vi "Read Data as Bytes.vi"(7 "Read Image Size (Default: T)":bool=TRUE, 8 "error in (no error)":errorcluster, 11 "Buffer in":refnum<class "Buffer.lvclass">) -> (0 "error out":errorcluster, 1 "Image Size":T1, 2 "Data":u8[](array[numeric]), 3 "Buffer":refnum<class "Buffer.lvclass">)   [LabVIEW 2020, in "Buffer.lvclass"]
uses:
  Buffer.lvclass
  Image Size.ctl
  Buffer.lvclass/Buffer.ctl
  GetBufferImageDimensions.vi
  <vilib>/Utility/error.llb/Error Cluster From Error Code.vi
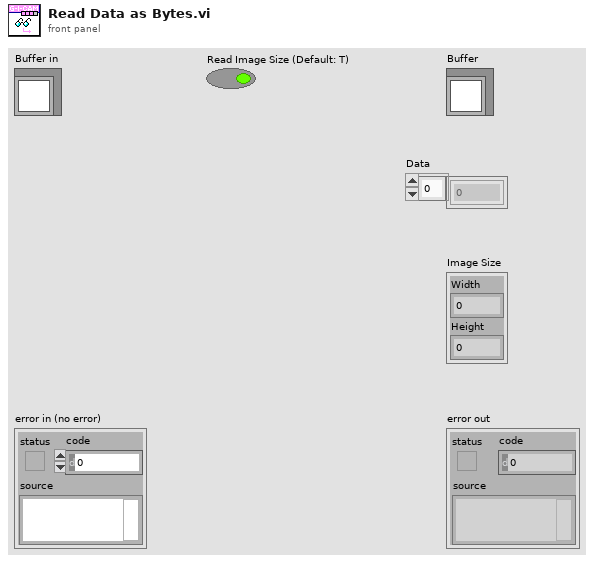
[diagram p1: front panel]
types:
  T1 = typedef "Buffer.lvclass/Image Size.ctl" = cluster{"Width":u16, "Height":u16}
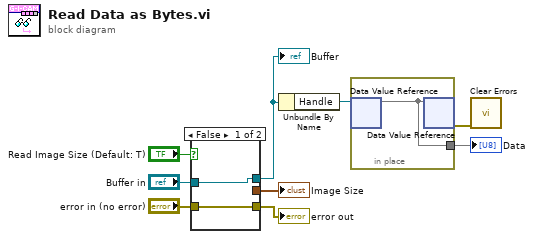
[diagram p0: block diagram]
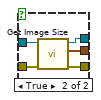
[diagram p2: hidden frame]
diagram:
  n1 = case shown="False" "Read Image Size (Default: T)" {
    tunnel: [w10 w16] -> w8
    tunnel: "Buffer in" -> [w11 w15]
    tunnel: "error in (no error)" -> [w10 w14]
    tunnel: [w11 w13] -> w5
    tunnel: [_ w12] -> w2
    frame False {
    }
    frame True {
      n2 = call "Get Image Size.vi"("error in (no error)"=w14, "Buffer in"=w15) -> ("error out"=w16:errorcluster, "Image Size"=w12:T1, "Buffer"=w13:refnum<class "Buffer.lvclass">)  [unwired: 7 in]
    }
  }
  "error out" <- w8
  "Buffer" <- w5
  "Image Size" <- w2
  n3 = Unbundle By Name(w5) -> ("Handle"=w4:refnum<data-value>)
  n4 = in-place {
    in-place-border: [w17] -> w9
    n5 = in-place-dvr #1(w4) -> (w17:u8[])  [unwired: 1 out]
    n6 = in-place-dvr #1(w17) -> (w3:errorcluster)  [unwired: 1 out]
  }
  "Data" <- w9
  n7 = call <vilib>:"Clear Errors.vi"("error in (no error)"=w3) -> ()  [unwired: 5 in, 2 out]
